vi "Get Default Instrument Configuration.vi"(0 "Instrument Handle In":refnum<k21>) -> (4 "Instrument Handle Out":refnum<k21>, 8 "SG Configuration":T1={"SelectedPorts"="", "Reference Clock Source"="PXI_CLK", "Carrier Frequency (Hz)"=1000000000.0, "DUT Average Input Power (dBm)"=-10.0, "External Attenuation (dB)"=0.0, "LO Sharing Mode"=enum."Automatic", "LO Routing Configurations"=[{"Channel Name"="", "Source"="Onboard", "Export Enabled"=FALSE}], "LO Offset Configuration"={"Mode"=enum."Automatic", "Offset (Hz)"=0.0}} {"LO Offset Configuration"."Offset (Hz)" format="%#_6p"; "Carrier Frequency (Hz)" format="%#_6p"})   [LabVIEW 2016, in "SG.lvlib"]
uses:
  SG.lvlib
  Instrument Configuration.ctl
  <instrlib>/niRFSG/niRFSG.llb/niRFSG Ref Clock Sources.ctl
  Common/Local Oscillator Sharing Mode.ctl
  Common/Local Oscillator Routing Configuration.ctl
  Common/Local Oscillator Frequency Offset Configuration.ctl
  Common/Local Oscillator Frequency Offset Mode.ctl
  <resource>/objmgr/RFmxInstr.rc
  Common/Common.lvlib
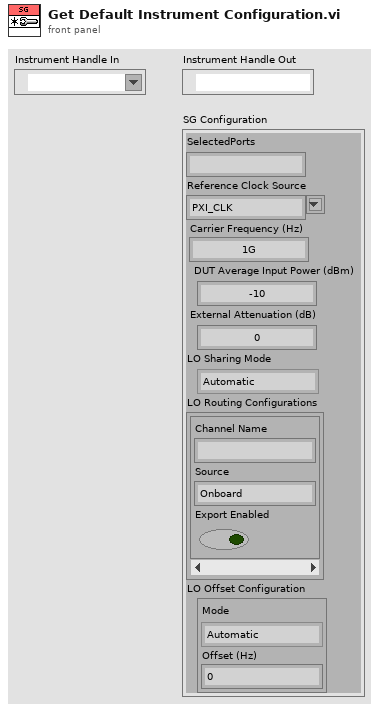
[diagram p1: front panel]
types:
  T1 = typedef "SG.lvlib/Instrument Configuration.ctl" = cluster{"SelectedPorts":string, "Reference Clock Source":T2, "Carrier Frequency (Hz)":dbl, "DUT Average Input Power (dBm)":dbl, "External Attenuation (dB)":dbl, "LO Sharing Mode":T3, "LO Routing Configurations":T4[], "LO Offset Configuration":T5}
  T2 = typedef "niRFSG Ref Clock Sources.ctl" = string
  T3 = typedef "Common.lvlib/Local Oscillator Sharing Mode.ctl" = enum16{"None", "Automatic", "Manual"}
  T4 = typedef "Common.lvlib/Local Oscillator Routing Configuration.ctl" = cluster{"Channel Name":string, "Source":string, "Export Enabled":bool}
  T5 = typedef "Common.lvlib/Local Oscillator Frequency Offset Configuration.ctl" = cluster{"Mode":T6, "Offset (Hz)":dbl}
  T6 = typedef "Common.lvlib/Local Oscillator Frequency Offset Mode.ctl" = enum16{"No Offset", "Automatic", "User Defined"}
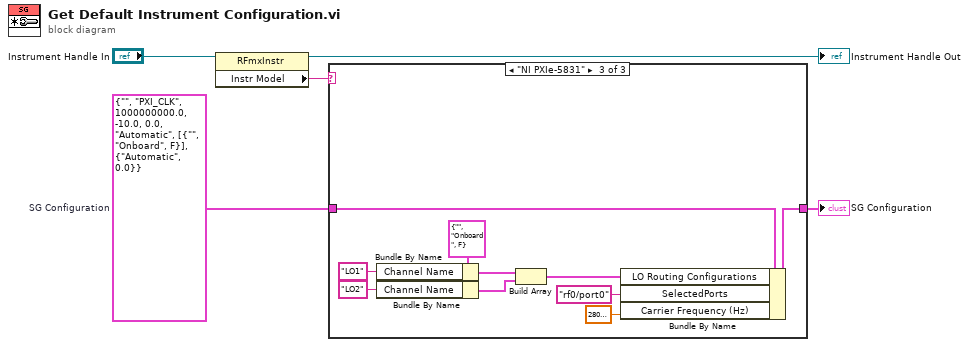
[diagram p0: block diagram]
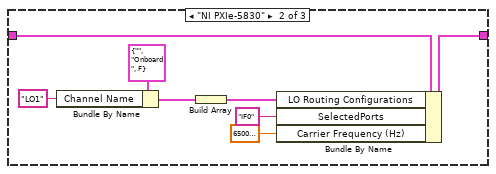
[diagram p3: hidden frame]
diagram:
  w1 = T1 {"SelectedPorts"="", "Reference Clock Source"="PXI_CLK", "Carrier Frequency (Hz)"=1000000000.0, "DUT Average Input Power (dBm)"=-10.0, "External Attenuation (dB)"=0.0, "LO Sharing Mode"=enum."Automatic", "LO Routing Configurations"=[{"Channel Name"="", "Source"="Onboard", "Export Enabled"=FALSE}], "LO Offset Configuration"={"Mode"=enum."Automatic", "Offset (Hz)"=0.0}}  # SG Configuration
  n1 = property class="RFmxInstr"(reference="Instrument Handle In") -> (reference out=→"Instrument Handle Out":refnum<k21>, "Instr Model"=w2:string)  [unwired: 1 in, 1 out]
  n2 = case shown="\"NI PXIe-5831\"" w2 {
    tunnel: w1 -> [w6 w13 w23]
    tunnel: [w6 w12 w22] -> w3
    frame Default {
    }
    frame "NI PXIe-5830" {
      n3 = Bundle By Name(cluster=T4 {"Channel Name"="", "Source"="Onboard", "Export Enabled"=FALSE} ("Local Oscillator Routing Configuration"), "Channel Name"="LO1") -> (w10:T4)
      n4 = Build Array(w10) -> (w9:T4[])
      n5 = Bundle By Name(cluster=w13, "LO Routing Configurations"=w9, "SelectedPorts"="IF0", "Carrier Frequency (Hz)"=6500000000.0) -> (w12:T1)
    }
    frame "NI PXIe-5831" {
      w24 = T4 {"Channel Name"="", "Source"="Onboard", "Export Enabled"=FALSE} ("Local Oscillator Routing Configuration")
      n6 = Bundle By Name(cluster=w24, "Channel Name"="LO1") -> (w19:T4)
      n7 = Bundle By Name(cluster=w24, "Channel Name"="LO2") -> (w18:T4)
      n8 = Build Array(w19, w18) -> (w17:T4[])
      n9 = Bundle By Name(cluster=w23, "LO Routing Configurations"=w17, "SelectedPorts"="rf0/port0", "Carrier Frequency (Hz)"=28000000000.0) -> (w22:T1)
    }
  }
  "SG Configuration" <- w3
